vi "Palette Cursors.vi"(8 "error in (no error)":errorcluster, 9 "Initialize":bool, 10 "Index":i32, 11 "Cursor IDs in":refnum<k1>[](array[refnum])) -> (0 "error out":errorcluster, 2 "cursor ID":refnum<k1>, 3 "Cursor IDs out":refnum<k1>[](array[refnum]))   [LabVIEW 2018]
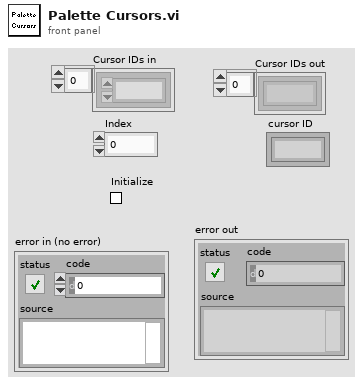
[diagram p1: front panel]
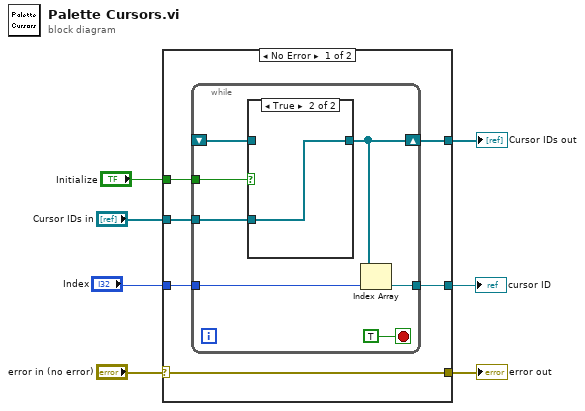
[diagram p0: block diagram]
diagram:
  n1 = case shown="No Error" "error in (no error)" {
    selector: "error in (no error)" -> [w13 w23]
    tunnel: [w13 w23] -> w6
    tunnel: [w12 _] -> w5
    tunnel: [w11 _] -> w4
    tunnel: "Index" -> [w10 _]
    tunnel: "Initialize" -> [w9 _]
    tunnel: "Cursor IDs in" -> [w8 _]
    frame No Error {
      n2 = while {
        shift-right: [w15] -> w12
        shift-left: _ -> [w18]
        tunnel: [w20] -> w11
        tunnel: w10 -> [w19]
        tunnel: w9 -> [w17]
        tunnel: w8 -> [w16]
        stop <- TRUE stop-if-true
        n3 = case shown="True" w17 {
          tunnel: w18 -> [w21 _]
          tunnel: w16 -> [_ w22]
          tunnel: [w21 w22] -> w15
          frame False {
          }
          frame True {
          }
        }
        n4 = Index Array(array=w15, index=w19) -> (element=w20:refnum<k1>)
      }
    }
    frame Error {
    }
  }
  "Cursor IDs out" <- w5
  "error out" <- w6
  "cursor ID" <- w4
